vi "참조 생성하기 1.vi"() -> ()   [LabVIEW 2020]
panel:
  in  "숫자형":dbl
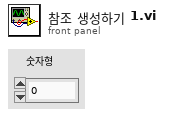
[diagram p1: front panel]
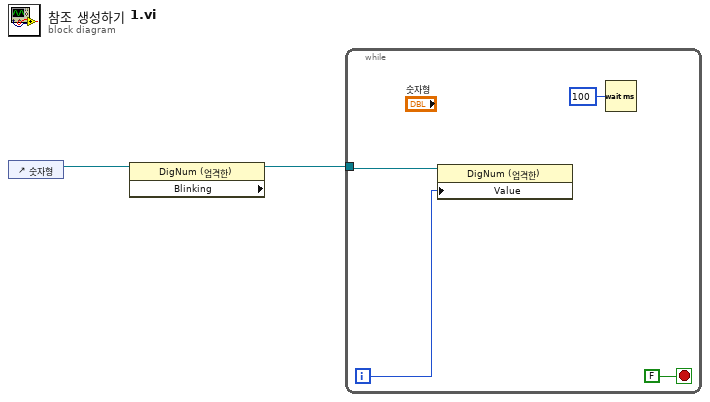
[diagram p0: block diagram]
diagram:
  n1 = control-ref of="숫자형"() -> (w2:refnum<vi>)
  n2 = property class="DigNum (엄격한)" props=["Blinking"](reference=w2) -> (reference out=w1:refnum<vi>)  [unwired: 1 in, 2 out]
  n3 = while {
    tunnel: w1 -> [w6]
    i -> [w5]
    stop <- FALSE stop-if-true
    n4 = property class="DigNum (엄격한)"(reference=w6, "Value"=w5) -> ()  [unwired: 1 in, 2 out]
    n5 = Wait (ms)(milliseconds to wait=u32 100 ("대기 시간 (ms)")) -> ()  [unwired: 1 out]
  }
